vi "Forward Pass [1.1.0.0].vi"(0 "x[t]":T1=[[0.0], [1.0], [0.0]], 2 "h[t-1]":T1=[[0.9], [0.1]], 5 "params":cluster{"Wxq":T1, "Whq":T1, "bq":T1}={"Wxq"=[[0.57813, 2.5697, -0.0219857], [-2.4696, -0.172737, 2.44961362]], "Whq"=[[-1.39960002, 0.96174453], [0.36456552, -0.47706397]], "bq"=[[0.5353143], [-1.98598657]]}, 7 "Activation":enum16{"sigmoid", "tanh", "ReLU", "Identity"}(ring)=enum."tanh") -> (16 "Vector":T1=[[0.9596566296381405], [-0.9543425350839243]])   [LabVIEW 2014]
uses:
  <vilib>/Analysis/Matrix/Datatypes/RealMatrix.ctl
  <vilib>/Analysis/baseanly.llb/Real A x B.vi
  <vilib>/Analysis/Matrix/Numeric/Add/Add - RM,RM.vi
  <vilib>/Analysis/NI_AALBase.lvlib
  <vilib>/Analysis/Matrix/NI_Matrix.lvlib
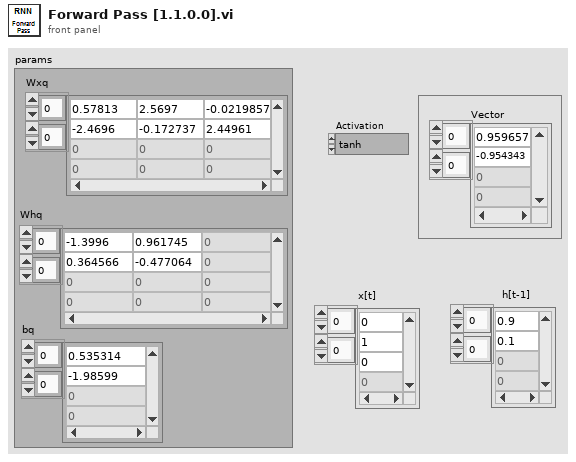
[diagram p1: front panel]
types:
  T1 = typedef "NI_Matrix.lvlib/RealMatrix.ctl" = dbl[][]
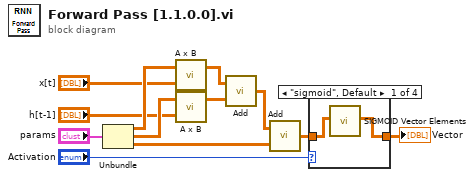
[diagram p0: block diagram]
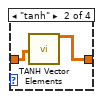
[diagram p2: hidden frame]
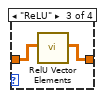
[diagram p3: hidden frame]
diagram:
  n1 = Unbundle("params") -> ("Wxq"=w8:T1, "Whq"=w9:T1, "bq"=w2:T1)
  n2 = call-poly <vilib>:"A x B.vi"("B"="x[t]", "A"=w8) -> ("A x B"=w12:T1)  [unwired: 1 out]
  n3 = call-poly <vilib>:"A x B.vi"("B"="h[t-1]", "A"=w9) -> ("A x B"=w11:T1)  [unwired: 1 out]
  n4 = call-poly <vilib>:"Add.vi"("Real Matrix B"=w11, "Real Matrix A"=w12) -> ("A + B"=w1:T1)
  n5 = call-poly <vilib>:"Add.vi"("Real Matrix B"=w2, "Real Matrix A"=w1) -> ("A + B"=w4:T1)
  n6 = case shown="\"sigmoid\", Default" "Activation" {
    tunnel: w4 -> [w13 w15 w17 w19]
    tunnel: [w14 w16 w18 w19] -> w3
    frame "sigmoid", Default {
      n7 = call "SIGMOID Vector Elements.vi"("X"=w13) -> ("sigmoid(X)"=w14:T1)  [unwired: 18 in]
    }
    frame "tanh" {
      n8 = call "TANH Vector Elements.vi"("X"=w15) -> ("tanh(X)"=w16:T1)  [unwired: 18 in]
    }
    frame "ReLU" {
      n9 = call "RelU Vector Elements.vi"("X"=w17) -> ("RelU(X)"=w18:T1)  [unwired: 18 in]
    }
    frame "Identity" {
    }
  }
  "Vector" <- w3
